vi "Plotter FGV Cluster.vi"(8 "error in":errorcluster, 10 "Function":enum16{"Read", "Write", "Clear"}(ring), 11 "Cluster in":T1={"Multicast Address"="234.5.6.9", "Plotter Busy"=FALSE, "Plotter Exit"=FALSE, "Mcast Port"=58449}) -> (0 "error out":errorcluster, 3 "Cluster out":T1={"Multicast Address"="234.5.6.9", "Plotter Busy"=FALSE, "Plotter Exit"=FALSE, "Mcast Port"=58449})   [LabVIEW 2013]
uses:
  Plotter FGV cluster control.ctl
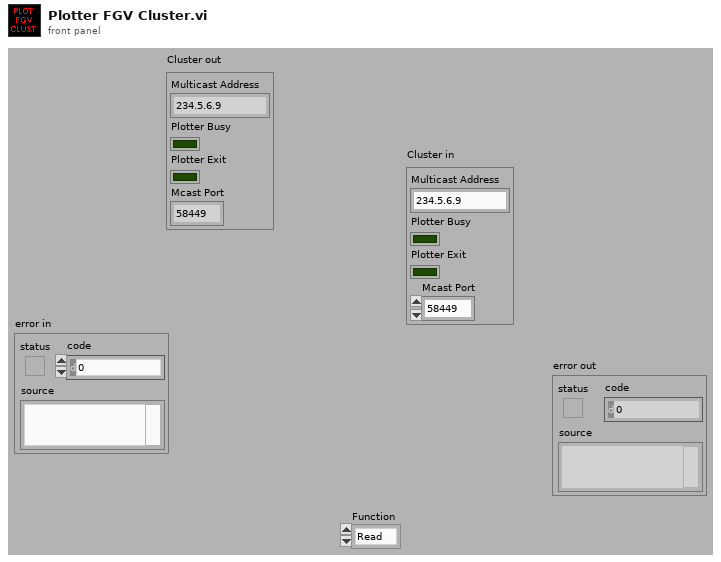
[diagram p1: front panel]
types:
  T1 = typedef "Plotter FGV cluster control.ctl" = cluster{"Multicast Address":string, "Plotter Busy":bool, "Plotter Exit":bool, "Mcast Port":u16}
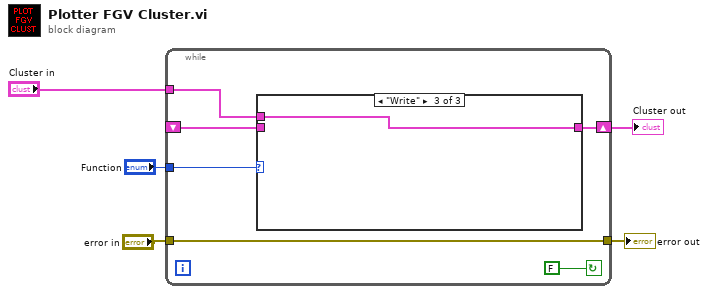
[diagram p0: block diagram]
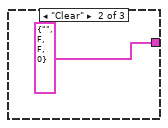
[diagram p3: hidden frame]
diagram:
  n1 = while {
    shift-right: [w9] -> w1
    shift-left: _ -> [w8]
    tunnel: "Function" -> [w11]
    tunnel: "Cluster in" -> [w10]
    tunnel: "error in" -> [w6]
    tunnel: [w6] -> w3
    stop <- FALSE continue-if-true
    n2 = case shown="\"Write\"" w11 {
      tunnel: w10 -> [_ _ w14]
      tunnel: [w12 T1 {"Multicast Address"="", "Plotter Busy"=FALSE, "Plotter Exit"=FALSE, "Mcast Port"=0} ("Cluster in") w14] -> w9
      tunnel: w8 -> [w12 _ _]
      frame "Read", Default {
      }
      frame "Clear" {
      }
      frame "Write" {
      }
    }
  }
  "error out" <- w3
  "Cluster out" <- w1
